vi "Meas (SubVI).vi"(9 "Param":T1 {"FChB" format="%_4p"; "FChA" format="%_4p"}, 11 "Array in":waveform(dbl)[](array[waveform])) -> (2 "RMS,mV":dbl[](array[numeric]), 3 "Freq":dbl[](array[numeric]))   [LabVIEW 2017]
uses:
  <vilib>/measure/matone.llb/Extract Single Tone Information 1 Chan.vi
  <vilib>/measure/NI_MAPro.lvlib
panel:
  out "error out":errorcluster
  in  "error in":errorcluster
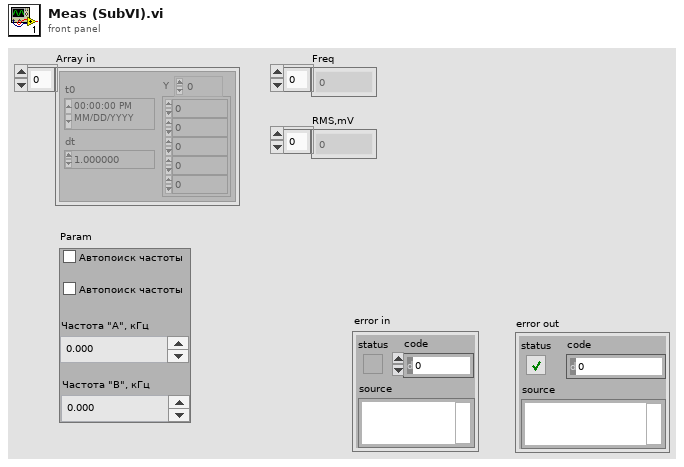
[diagram p1: front panel]
types:
  T1 = cluster{"AutoFindFreqChA":bool, "AutoFindFreqChB":bool, "FChA":dbl, "FChB":dbl}
  T2 = cluster{"approx freq. (optional)":dbl, "search (+/- % of Fsampl.)":dbl}
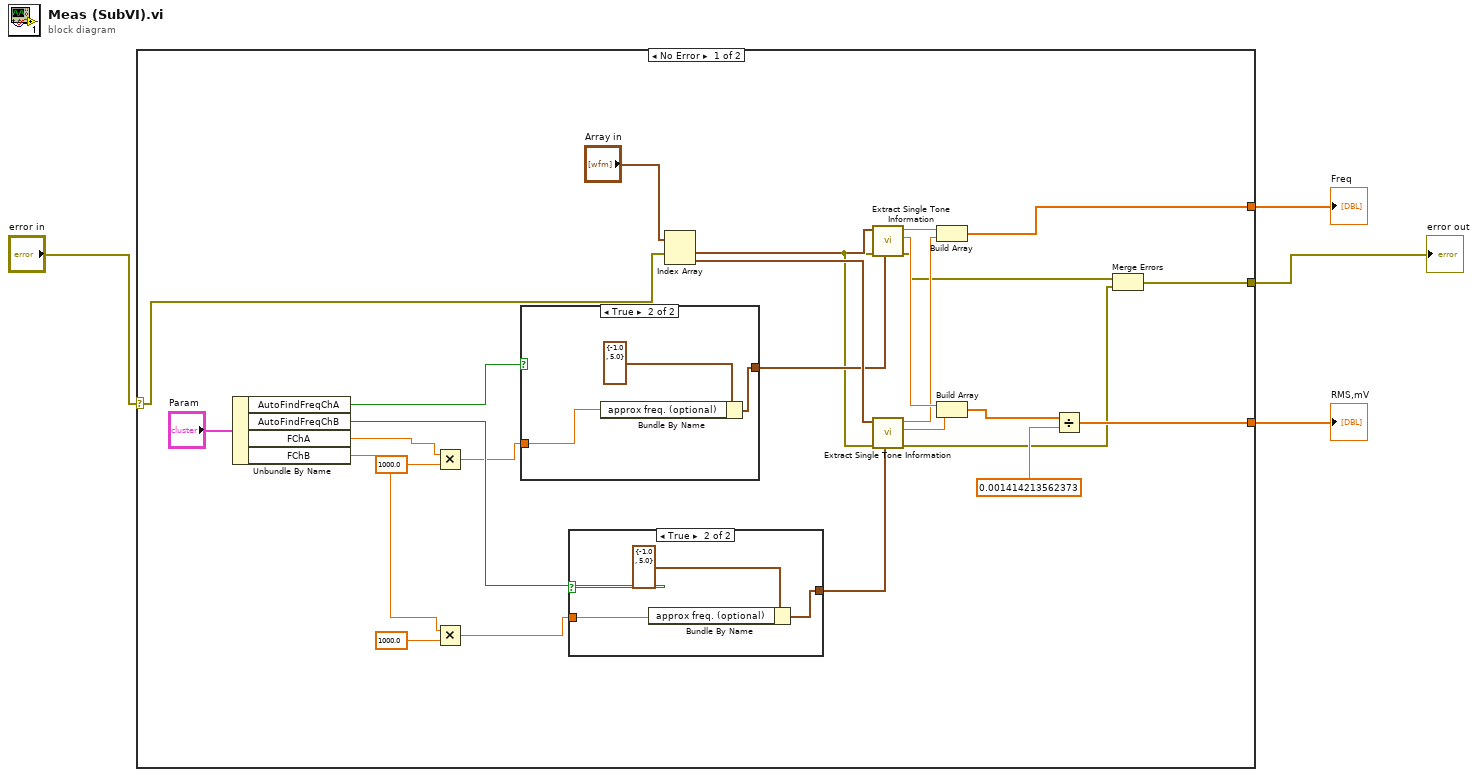
[diagram p0: block diagram]
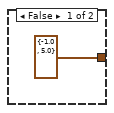
[diagram p2: hidden frame]
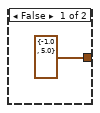
[diagram p3: hidden frame]
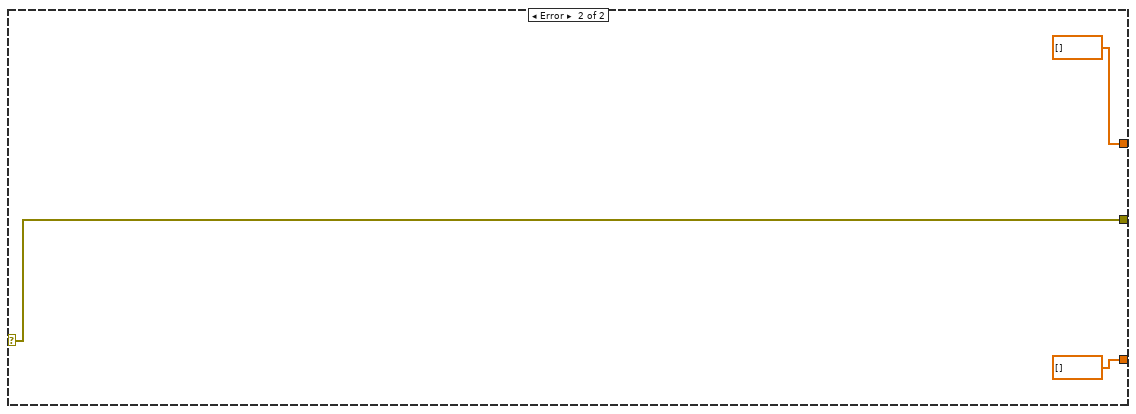
[diagram p4: hidden frame]
diagram:
  n1 = case shown="No Error" "error in" {
    selector: "error in" -> [w12 w41]
    tunnel: [w30 dbl[] []] -> w4
    tunnel: [w21 dbl[] []] -> w3
    tunnel: [w11 w41] -> w1
    frame No Error {
      n2 = Unbundle By Name("Param") -> ("AutoFindFreqChA"=w16:bool, "AutoFindFreqChB"=w15:bool, "FChA"=w10:dbl, "FChB"=w6:dbl)
      n3 = Multiply(x=w10, y=1000.0) -> (x*y=w8:dbl)
      n4 = Multiply(x=w6, y=1000.0) -> (x*y=w5:dbl)
      n5 = case shown="True" w16 {
        tunnel: [T2 {"approx freq. (optional)"=-1.0, "search (+/- % of Fsampl.)"=5.0} ("advanced search") w33] -> w18
        tunnel: w8 -> [_ w32]
        frame False {
        }
        frame True {
          n6 = Bundle By Name(cluster=T2 {"approx freq. (optional)"=-1.0, "search (+/- % of Fsampl.)"=5.0} ("advanced search"), "approx freq. (optional)"=w32) -> (w33:T2)
        }
      }
      n7 = case shown="True" w15 {
        tunnel: [T2 {"approx freq. (optional)"=-1.0, "search (+/- % of Fsampl.)"=5.0} ("advanced search") w37] -> w19
        tunnel: w5 -> [_ w36]
        frame False {
        }
        frame True {
          n8 = Bundle By Name(cluster=T2 {"approx freq. (optional)"=-1.0, "search (+/- % of Fsampl.)"=5.0} ("advanced search"), "approx freq. (optional)"=w36) -> (w37:T2)
        }
      }
      n9 = Index Array(array="Array in") -> (element #1=w23:waveform(dbl), element #2=w24:waveform(dbl))  [unwired: 2 in]
      n10 = call-poly <vilib>:"Extract Single Tone Information.vi"("advanced search"=w18, "error in (no error)"=w12, "time signal in"=w23) -> ("error out"=w13:errorcluster, "detected amplitude"=w27:dbl, "detected frequency"=w25:dbl)  [unwired: 3 in, 3 out]
      n11 = call-poly <vilib>:"Extract Single Tone Information.vi"("advanced search"=w19, "error in (no error)"=w12, "time signal in"=w24) -> ("error out"=w14:errorcluster, "detected amplitude"=w28:dbl, "detected frequency"=w26:dbl)  [unwired: 3 in, 3 out]
      n12 = Build Array(w25, w26) -> (w30:dbl[])
      n13 = Build Array(w27, w28) -> (w29:dbl[])
      n14 = Divide(x=w29, y=0.001414213562373) -> (x/y=w21:dbl[])
      n15 = Merge Errors(w13, w14) -> (w11:errorcluster)
    }
    frame Error {
    }
  }
  "Freq" <- w4
  "RMS,mV" <- w3
  "error out" <- w1
